vi "ReadObjectLayout.vi"(7 "properties to ignore":variant, 8 "error in (no error)":errorcluster, 10 "GObj Refnum":refnum<vi>, 11 "Array Control Layout in":refnum<class "Array Control Layout.lvclass">) -> (0 "error out":errorcluster, 3 "Array Control Layout out":refnum<class "Array Control Layout.lvclass">)   [LabVIEW 2010, in "NI_SE_Front Panel Layout.lvlib" / "Array Control Layout.lvclass"]
doc: "Read layout information from the GObj Refnum."
uses:
  Array Control Layout.lvclass
  Control Layout/Control Layout.lvclass
  Array Control Layout.lvclass/Array Control Layout.ctl
  NI_SE_Front Panel Layout.lvlib
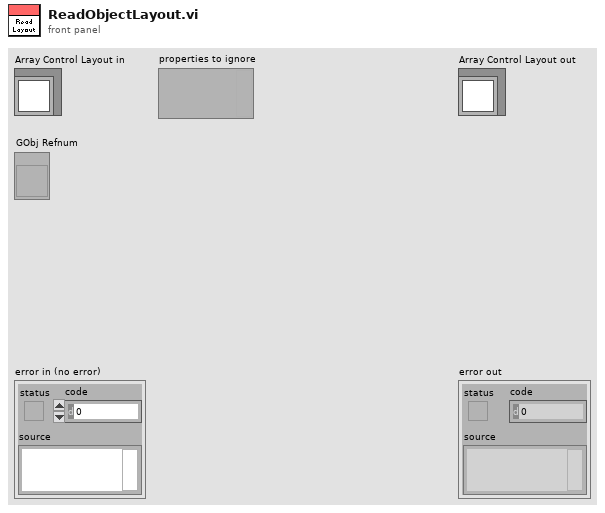
[diagram p1: front panel]
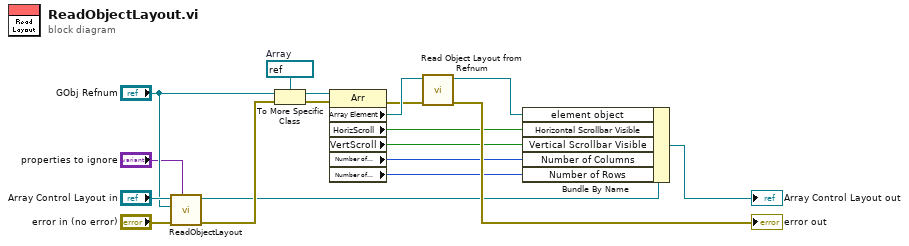
[diagram p0: block diagram]
diagram:
  w10 = refnum<vi> refnum  # Array
  n1 = call-parent "ReadObjectLayout.vi"("properties to ignore"="properties to ignore", "error in (no error)"="error in (no error)", "GObj Refnum"="GObj Refnum", "Control Layout in"="Array Control Layout in") -> ("error out"=w16:errorcluster, "Control Layout out"=w14:refnum<class "Array Control Layout.lvclass">)  [unwired: 6 in]
  n2 = To More Specific Class(target class=w10, reference="GObj Refnum", error in=w16) -> (specific class reference=w9:refnum<vi>, error out=w8:errorcluster)
  n3 = property class="Arr"(reference=w9, error in=w8) -> (error out=w1:errorcluster, "Array Element"=w3:refnum<vi>, "HorizScroll"=w7:bool, "VertScroll"=w6:bool, "Number of Columns"=w5:u32, "Number of Rows"=w4:u32)  [unwired: 1 out]
  n4 = call "Read Object Layout from Refnum.vi"("error in"=w1, "GObj refnum"=w3) -> ("error out"=→"error out":errorcluster, "object layout"=w2:refnum<class "Object Layout.lvclass">)  [unwired: 7 in, 1 out]
  n5 = Bundle By Name(cluster=w14, "element object"=w2, "Horizontal Scrollbar Visible"=w7, "Vertical Scrollbar Visible"=w6, "Number of Columns"=w5, "Number of Rows"=w4) -> (→"Array Control Layout out":refnum<class "Array Control Layout.lvclass">)
